vi "Overlay Circle.vi"(10 "Circles (Shape Detection 1) in":T1(array[cluster]), 11 "Refnum in":T2) -> (1 "Position":cluster{"X":sgl, "Y":sgl}, 2 "Circles (Shape Detection 1) out":T1(array[cluster]) {"Position"."Y" format="%.2f"; "Position"."X" format="%.2f"}, 3 "Refnum out":T2)   [LabVIEW 2015]
uses:
  <vilib>/vision/Image Controls.llb/IMAQ Image.ctl
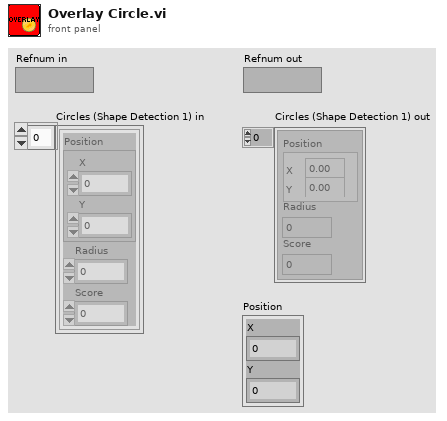
[diagram p1: front panel]
types:
  T1 = cluster{"Position":cluster{"X":sgl, "Y":sgl}, "Radius":dbl, "Score":dbl}[]
  T2 = typedef "IMAQ Image.ctl" = refnum<image>
  T3 = cluster{"Circles (Shape Detection 1) in[0]":cluster{"Position":cluster{"X":sgl, "Y":sgl}, "Radius":dbl, "Score":dbl}, "Circles (Shape Detection 1) in[1]":cluster{"Position":cluster{"X":sgl, "Y":sgl}, "Radius":dbl, "Score":dbl}, "Circles (Shape Detection 1) in[2]":cluster{"Position":cluster{"X":sgl, "Y":sgl}, "Radius":dbl, "Score":dbl}, "Circles (Shape Detection 1) in[3]":cluster{"Position":cluster{"X":sgl, "Y":sgl}, "Radius":dbl, "Score":dbl}, "Circles (Shape Detection 1) in[4]":cluster{"Position":cluster{"X":sgl, "Y":sgl}, "Radius":dbl, "Score":dbl}, "Circles (Shape Detection 1) in[5]":cluster{"Position":cluster{"X":sgl, "Y":sgl}, "Radius":dbl, "Score":dbl}, "Circles (Shape Detection 1) in[6]":cluster{"Position":cluster{"X":sgl, "Y":sgl}, "Radius":dbl, "Score":dbl}, "Circles (Shape Detection 1) in[7]":cluster{"Position":cluster{"X":sgl, "Y":sgl}, "Radius":dbl, "Score":dbl}, "Circles (Shape Detection 1) in[8]":cluster{"Position":cluster{"X":sgl, "Y":sgl}, "Radius":dbl, "Score":dbl}}
  T4 = cluster{"Position":cluster{"X":sgl, "Y":sgl}, "Radius":dbl, "Score":dbl}
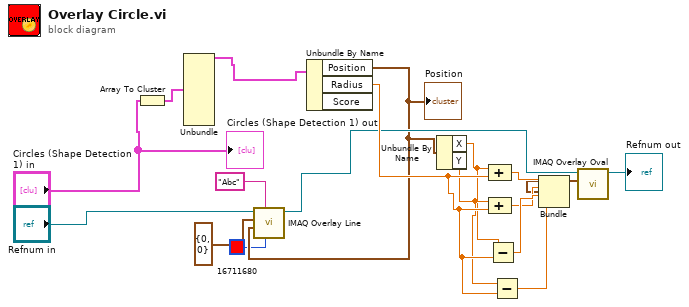
[diagram p0: block diagram]
diagram:
  n1 = Array To Cluster(array="Circles (Shape Detection 1) in") -> (cluster=w2:T3)
  n2 = Unbundle(w2) -> ("Circles (Shape Detection 1) in[0]"=w3:T4)  [unwired: 8 out]
  n3 = Unbundle By Name(w3) -> ("Position"=w8:cluster{"X":sgl, "Y":sgl}, "Radius"=w17:dbl)  [unwired: 1 out]
  "Position" <- w8
  n4 = call "IMAQ Overlay Line"("Color"=u32 16711680, "Group"="Abc", "End Point"=w8, "Start Point"=cluster{"X":i32, "Y":i32} {"X"=0, "Y"=0}, "Image"="Refnum in") -> ("Image Out"=w10:T2)  [unwired: 5 in, 1 out]
  n5 = Unbundle By Name(w8) -> ("X"=w14:sgl, "Y"=w16:sgl)
  n6 = Subtract(x=w14, y=w17) -> (x-y=w15:dbl)
  n7 = Compound Arithmetic op=ADD(w14, w17) -> (w12:dbl)
  n8 = Compound Arithmetic op=ADD(w16, w17) -> (w13:dbl)
  n9 = Subtract(x=w16, y=w17) -> (x-y=w18:dbl)
  n10 = Bundle(w12, w13, w15, w18) -> (w11:cluster{dbl, dbl, dbl, dbl})  [unwired: 1 in]
  n11 = call "IMAQ Overlay Oval"("Bounding Rectangle"=w11, "Image"=w10) -> ("Image Out"=→"Refnum out":T2)  [unwired: 8 in, 1 out]
  "Circles (Shape Detection 1) out" <- "Circles (Shape Detection 1) in"
